vi "PlotHistgramAndProfile.vi"(8 "error in (no error)":errorcluster, 11 "Histgram":refnum<notifier>) -> (0 "error out":errorcluster)   [LabVIEW 2020, in "DisplayerUI.lvlib" / "DisplayerUI.lvclass"]
uses:
  DisplayerUI.lvclass
panel:
  in  "Live":bool
  in  "Exit":bool
  out "Profile":cluster{"X":dbl, "Y":dbl}[](graph)
  out "Histgram":cluster{"X":dbl, "Y":dbl}[](graph)
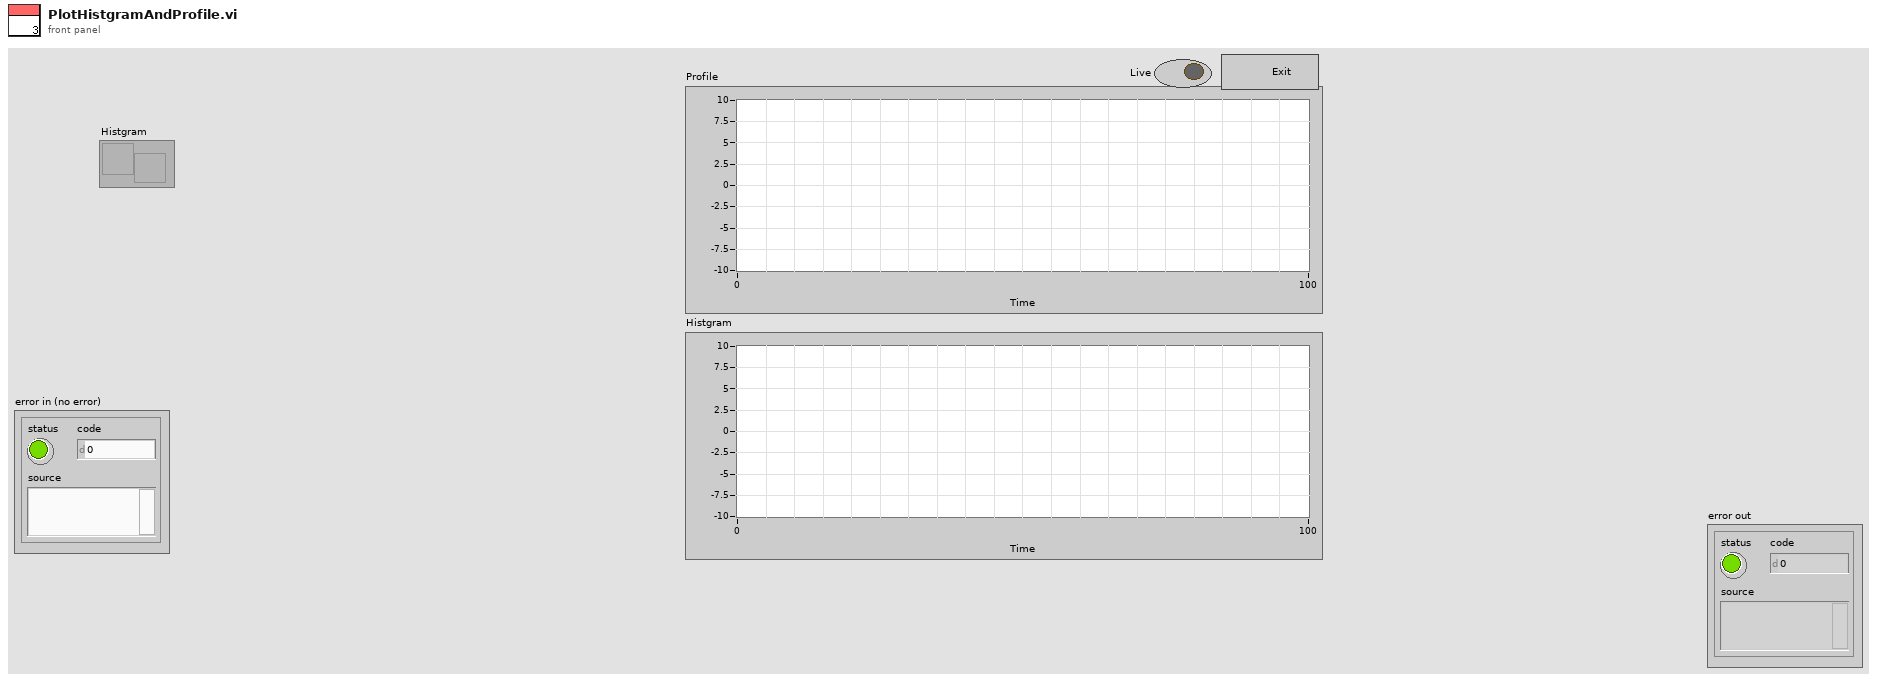
[diagram p1: front panel]
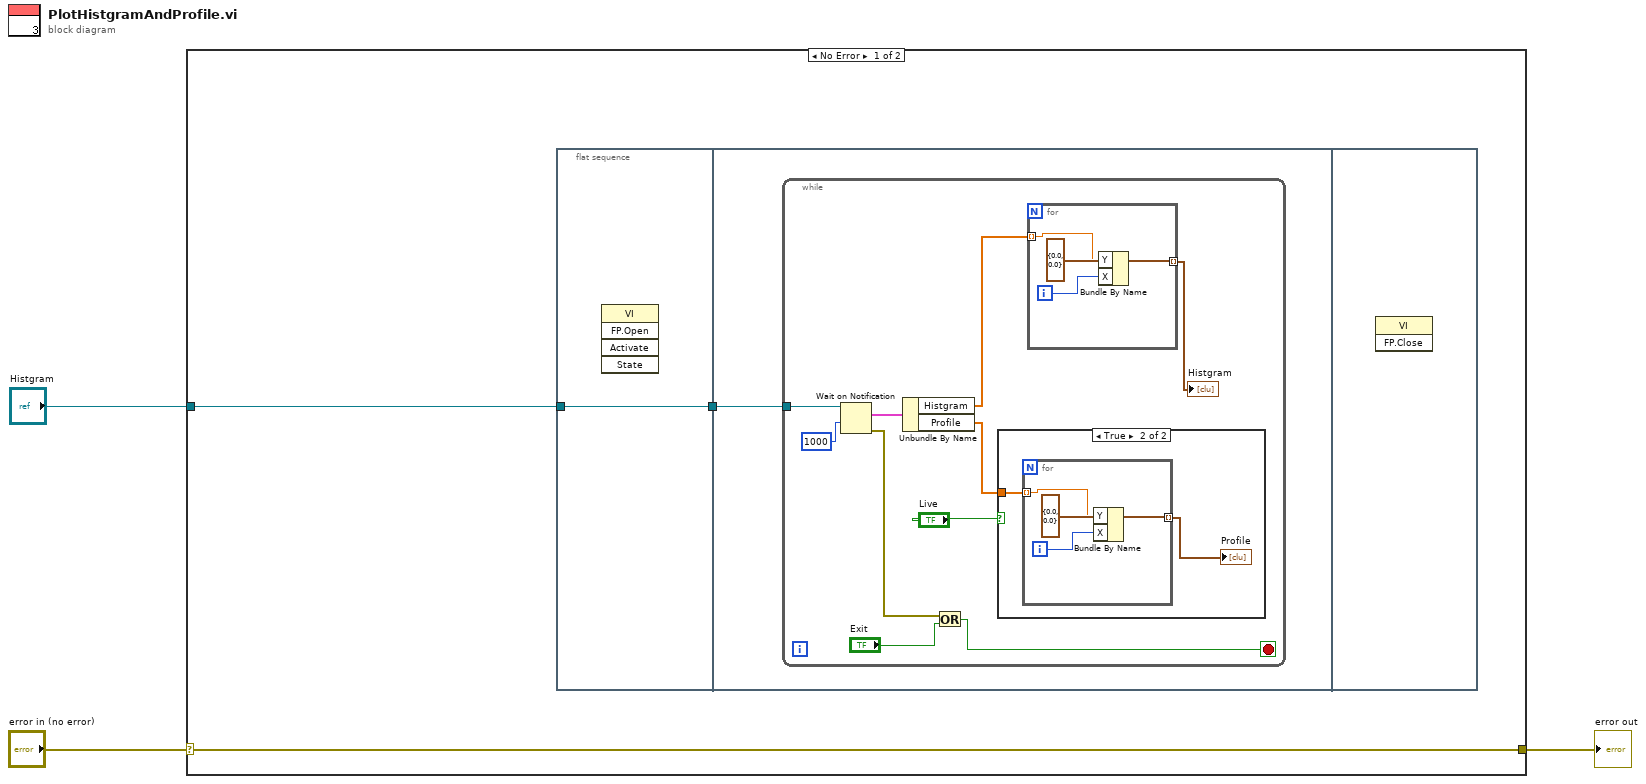
[diagram p0: block diagram]
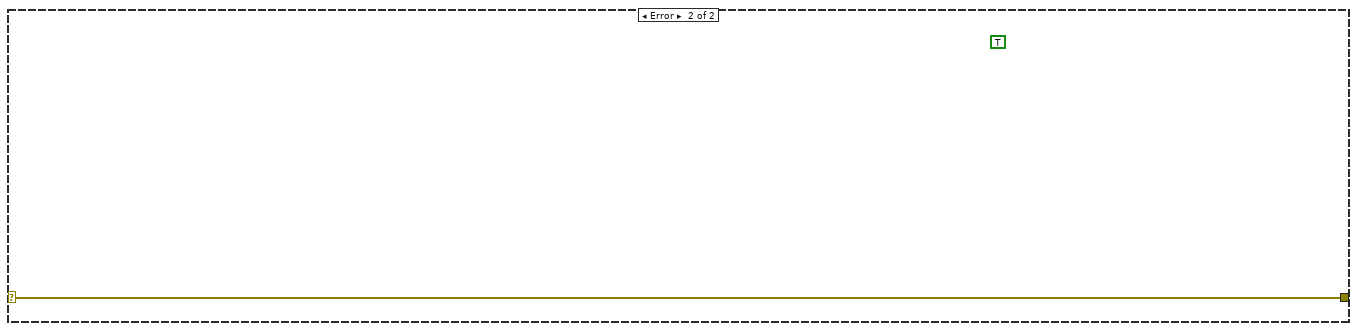
[diagram p3: hidden frame]
diagram:
  n1 = case shown="No Error" "error in (no error)" {
    selector: "error in (no error)" -> [w6 w29]
    tunnel: [w6 w29] -> w2
    tunnel: "Histgram" -> [w5 _]
    frame No Error {
      n2 = flat-sequence {
        tunnel: w5 -> [w7]
        tunnel: [w7] -> w4
        tunnel: w4 -> [w8]
        frame #0 {
          n3 = invoke class="VI" method="FP.Open"() -> ()  [unwired: 5 in, 5 out]
        }
        frame #1 {
          n4 = while {
            tunnel: w8 -> [w18]
            stop <- w11 stop-if-true
            n5 = Wait on Notification(notifier=w18, timeout in ms (-1)=1000) -> (notification=w17:cluster{"Histgram":dbl[], "Profile":dbl[]}, error out=w10:errorcluster)  [unwired: 2 in, 2 out]
            n6 = Unbundle By Name(w17) -> ("Histgram"=w15:dbl[], "Profile"=w14:dbl[])
            n7 = Or(x=w10, y="Exit") -> (x .or. y?=w11:bool)
            n8 = case shown="True" "Live" {
              tunnel: w14 -> [_ w19]
              frame False {
              }
              frame True {
                n9 = for {
                  tunnel: w19 -> [w21] mode=indexing
                  tunnel: [w23] -> w20 mode=indexing
                  i -> [w22]
                  n10 = Bundle By Name(cluster=cluster{"X":dbl, "Y":dbl} {"X"=0.0, "Y"=0.0}, "Y"=w21, "X"=w22) -> (w23:cluster{"X":dbl, "Y":dbl})
                }
                "Profile" <- w20
              }
            }
            n11 = for {
              tunnel: w15 -> [w25] mode=indexing
              tunnel: [w27] -> w16 mode=indexing
              i -> [w26]
              n12 = Bundle By Name(cluster=cluster{"X":dbl, "Y":dbl} {"X"=0.0, "Y"=0.0}, "Y"=w25, "X"=w26) -> (w27:cluster{"X":dbl, "Y":dbl})
            }
            "Histgram" <- w16
          }
        }
        frame #2 {
          n13 = invoke class="VI" method="FP.Close"() -> ()  [unwired: 3 in, 3 out]
        }
      }
    }
    frame Error {
      (unwired) TRUE ("UI Refresh Needed?")
    }
  }
  "error out" <- w2
